vi "save_testConditions.vi"(8 "error in (no error)":errorcluster, 11 "cmd":T5) -> (0 "error out":errorcluster)   [LabVIEW 2019]
uses:
  cmd_TestParaSave.ctl
  type_testpara.ctl
  Capacitor/cap_config.ctl
  Capacitor/Judge_RC.ctl
  _ctrl/rw.ctl
  Global_params.vi
  Global 1.vi
  <vilib>/Utility/xml.llb/Write to XML File(string).vi
  <vilib>/Utility/xml.llb/Read From XML File(string).vi
  SubVIs/common/Glob_Ref.vi
panel:
  out "Test Mode":T1
  out "RC-Testconfig.Test Mode":T1
  out "TestConditons":T2={"Breakdown-Spec"={"제어단 단선 Irms[mA](이하)"=0.0, "제어단 특성 전류 Irms[mA] Max"=0.0, "제어단 특성 전류 Irms[mA] Min"=0.0, "출력단 단선 Irms[mA](이하)"=0.0, "출력단 특성 전류 Irms[mA]  Max"=0.0, "출력단 특성전류 Irms[mA]  Min"=0.0, "온도[degree]"=0.0}, "RC-Testconfig"={"Test Mode"=enum."6.3.2 저온 작동/방치 시험", "ON time[ms]"=500.0, "OFF time[ms]"=500.0, "1. 작동시간[분]"=10000.0, "2. 미작동시간[분]"=10000.0, "3. 작동시간[분]"=10000.0, "level[V]"=12.0, "duty"=20.0, "Freq"=1.0, "Voltage+[V]"=20.0, "Voltage-[V]"=-20.0, "Current+[A]"=5.0, "Current-[A]"=-5.0, "출력전압[V]"=0.0, "출력전류[A]"=0.0, "OVP Level"=0.0, "OCP Level"=0.0, "Time Div"=7, "Record Len"=4, "방전 기준[V]"=0.0, "Repeate (Each Ch)"=1, "Cycle[N]"=1, "작동간격[분]"=10000.0, "TrigPos[%]"=0.0, "시험시간[분]"=1.0}, "RC-Test Judgement "={"전압 63%[mS] Min"=0.0, "전압 98%[mS] Min"=0.0, "전류 37%[mS] Min"=0.0, "접촉저항[mOhm] Min"=0.0, "출력전류 Irms[mA] Min"=0.0, "전압 63%[mS] Max"=0.0, "전압 98%[mS] Max"=0.0, "전류 37%[mS] Max"=0.0, "접촉저항[mOhm] Max"=0.0, "출력전류 Irms[mA] Max"=0.0}, "Log path"=path "", "file renew[Hr]"=0, "시험명"="R", "시험모드 선택"=enum."6.3.2 저온 작동/방치 시험"} {"RC-Testconfig"."시험시간[분]" min=1.0; "RC-Testconfig"."작동간격[분]" min=1.0; "RC-Testconfig"."3. 작동시간[분]" min=1.0; "RC-Testconfig"."2. 미작동시간[분]" min=1.0; "RC-Testconfig"."1. 작동시간[분]" min=1.0; "RC-Testconfig"."Time Div" items=["10m", "20ms", "50ms", "100ms", "200ms", "500ms", "1s", "2s", "5s", "10s", "20s", "30s", "1min", "2min", "5min"]; "RC-Testconfig"."OFF time[ms]" min=10000.0 max=1000000.0; "RC-Testconfig"."Current-[A]" min=-20.0 max=20.0 step=0.001; "RC-Testconfig"."Voltage-[V]" min=-115.0 max=115.0 step=0.01; "RC-Testconfig"."Current+[A]" min=0.0 max=60.0 step=0.01; "RC-Testconfig"."Voltage+[V]" min=0.0 max=120.0 step=0.1; "RC-Testconfig"."OCP Level" format="%#_13g"; "RC-Testconfig"."OVP Level" format="%#_13g"; "RC-Testconfig"."Record Len" items=["10k", "25k", "50k", "100k", "250k", "500k", "1M", "2.5M", "5M", "10M", "25M", "50M", "100M", "250M", "500M", "1G", "2G", "4G", "5G", "10G", "20G", "50G"]; "RC-Testconfig"."ON time[ms]" min=50.0 max=2000000.0}
  # "제어단"
  # "출력단"
  # "온도기준"
  # "제어단 전압"
  # "출력단 전원"
  # "DL950"
  # "Discharge"
  # "Test Cycle"
  # "작동 설정"
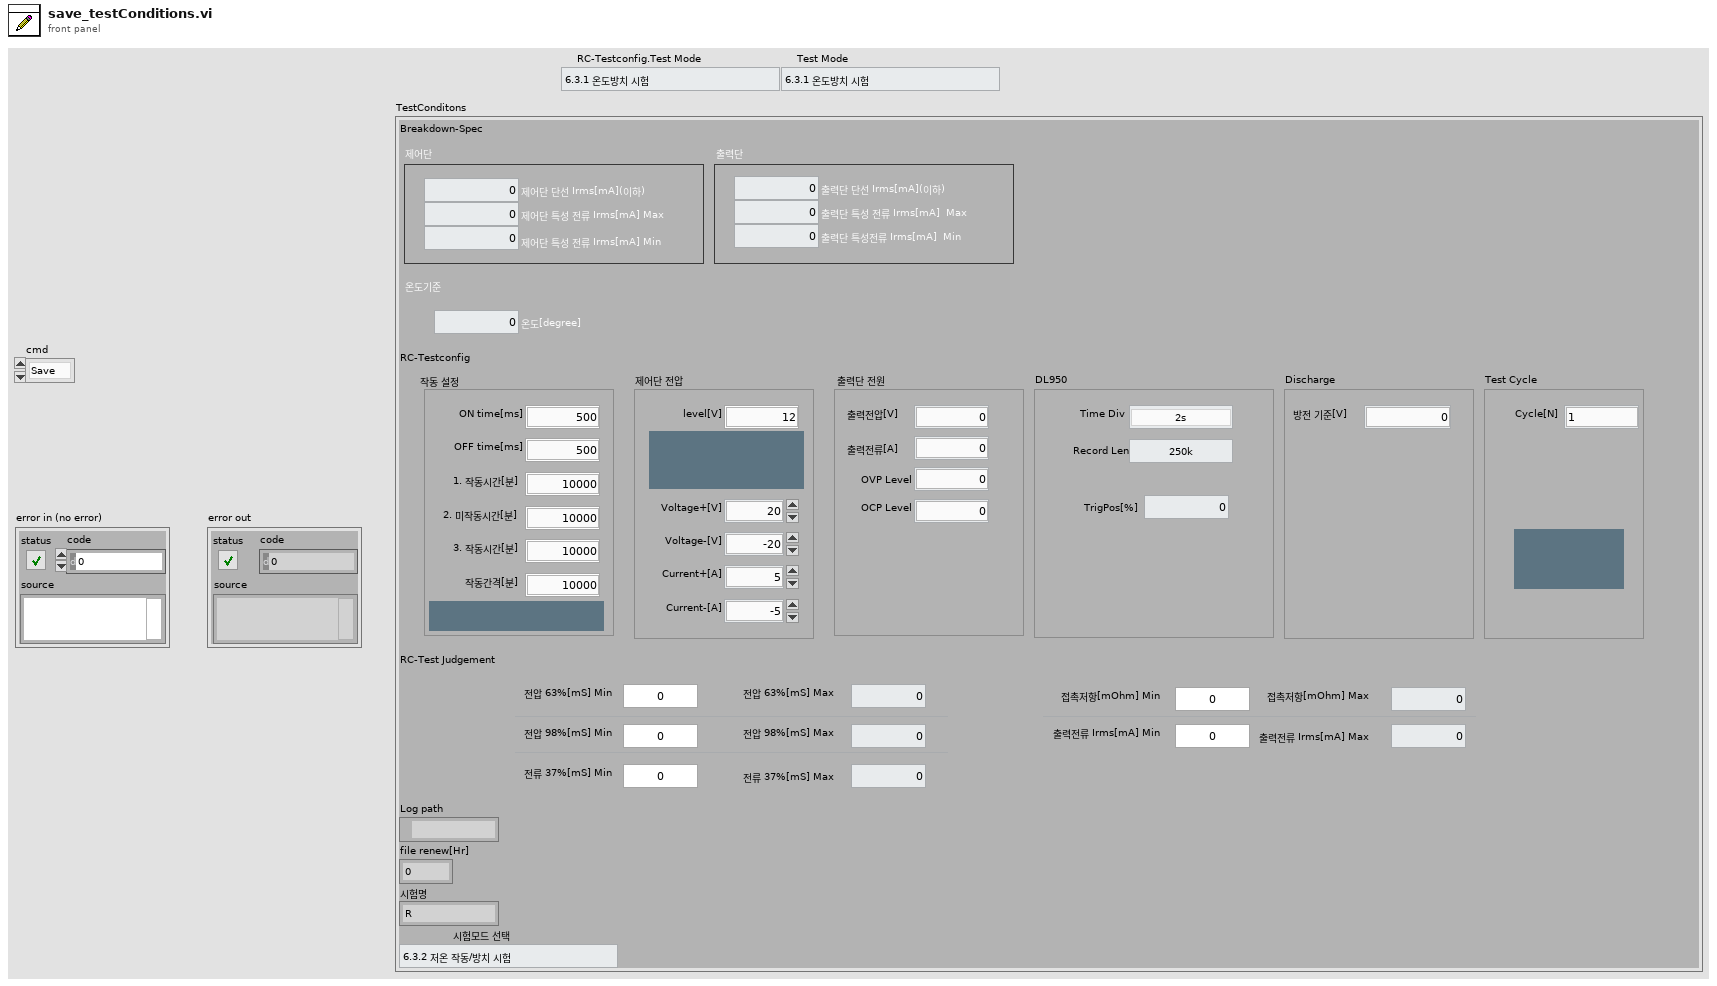
[diagram p1: front panel]
types:
  T1 = typedef "시험모드선택.ctl" = enum16{"6.3.1 온도방치 시험", "6.3.2 저온 작동/방치 시험", "6.3.3 고온 작동/방치 시험", "6.3.4 온도 싸이클 시험", "6.3.6 온습도 싸이클 시험", "6.3.7 고온고습 방치", "6.3.8 결로 시험", "6.3.9 빙결시험", "6.3.10 공진", "6.3.11.1 작동가진", "6.3.11.2 비작동 가진 ", "6.3.12 충격시험"}
  T2 = typedef "type_testpara.ctl" = cluster{"Breakdown-Spec":cluster{"제어단 단선 Irms[mA](이하)":dbl, "제어단 특성 전류 Irms[mA] Max":dbl, "제어단 특성 전류 Irms[mA] Min":dbl, "출력단 단선 Irms[mA](이하)":dbl, "출력단 특성 전류 Irms[mA]  Max":dbl, "출력단 특성전류 Irms[mA]  Min":dbl, "온도[degree]":dbl}, "RC-Testconfig":T3, "RC-Test Judgement ":T4, "Log path":path, "file renew[Hr]":u8, "시험명":string, "시험모드 선택":T1}
  T3 = typedef "cap_config.ctl" = cluster{"Test Mode":T1, "ON time[ms]":dbl, "OFF time[ms]":dbl, "1. 작동시간[분]":dbl, "2. 미작동시간[분]":dbl, "3. 작동시간[분]":dbl, "level[V]":dbl, "duty":dbl, "Freq":dbl, "Voltage+[V]":dbl, "Voltage-[V]":dbl, "Current+[A]":dbl, "Current-[A]":dbl, "출력전압[V]":dbl, "출력전류[A]":dbl, "OVP Level":dbl, "OCP Level":dbl, "Time Div":u16, "Record Len":i32, "방전 기준[V]":dbl, "Repeate (Each Ch)":u32, "Cycle[N]":u32, "작동간격[분]":dbl, "TrigPos[%]":dbl, "시험시간[분]":dbl}
  T4 = typedef "Judge_RC.ctl" = cluster{"전압 63%[mS] Min":dbl, "전압 98%[mS] Min":dbl, "전류 37%[mS] Min":dbl, "접촉저항[mOhm] Min":dbl, "출력전류 Irms[mA] Min":dbl, "전압 63%[mS] Max":dbl, "전압 98%[mS] Max":dbl, "전류 37%[mS] Max":dbl, "접촉저항[mOhm] Max":dbl, "출력전류 Irms[mA] Max":dbl}
  T5 = typedef "cmd_TestParaSave.ctl" = enum16{"Save", "Read", "Idle"}
  T6 = typedef "rw.ctl" = enum16{"read", "write"}
  T7 = enum16{"open", "replace", "create", "open or create", "replace or create", "replace or create with confirmation"}
  T8 = enum8{"Enabled", "Disabled", "Disabled and Grayed Out"}
  T9 = enum32{"6.3.2 저온 작동/방치 시험", "6.3.3 고온 작동/방치 시험", "6.3.4 온도 싸이클 시험", "6.3.6 온습도 싸이클 시험", "6.3.8 결로 시험", "6.3.9 빙결 시험"}
  T10 = cluster{"Freq":dbl, "level[V]":dbl, "duty":dbl, "On time[ms]":dbl}
  T11 = typedef "Test Mode.ctl" = enum32{"저항부하", "캐패시터부하", "B수명 - 1", "B수명 - 2", "B수명 - 3", "저전압모드 동작검사", "저전압모드 접촉저항", "고전압모드 동작검사"}
  T12 = typedef "ref_all.ctl" = cluster{"BP4610 Config":refnum<vi>, "DSP1950 Config":refnum<vi>, "2470-config":refnum<vi>, "cDAQ 9269 AO config":refnum<vi>, "cDAQ 9221 Config":refnum<vi>, "cDAQ-9467 Config":refnum<vi>, "Waveform":refnum<vi>, "DL950 wfm":refnum<vi>, "AI Graph":refnum<vi>, "AO_Wave-config":refnum<vi>, "DL950 items":refnum<vi>, "Volt":refnum<vi>, "Current":refnum<vi>, "AO_Level":refnum<vi>, "RC-Test Judgement ":refnum<vi>, "Log path":refnum<vi>, "시험명":refnum<vi>, "file renew[Hr]":refnum<vi>, "Breakdown-Spec":refnum<vi>, "paste":refnum<vi>, "copy":refnum<vi>, "DL950_config":refnum<vi>, "종료시간":refnum<vi>, "경과시간":refnum<vi>, "Apply":refnum<vi>, "DSP Config LV ":refnum<vi>, "Testconfig":refnum<vi>}
  T13 = typedef "Breakdown-Spec.ctl" = cluster{"제어단 단선 Irms[mA](이하)":dbl, "제어단 특성 전류 Irms[mA] Max":dbl, "제어단 특성 전류 Irms[mA] Min":dbl, "출력단 단선 Irms[mA](이하)":dbl, "출력단 특성 전류 Irms[mA]  Max":dbl, "출력단 특성전류 Irms[mA]  Min":dbl, "온도[degree]":dbl}
  T14 = cluster{"제어단 단선 Irms[mA](이하)":dbl, "제어단 특성 전류 Irms[mA] Max":dbl, "제어단 특성 전류 Irms[mA] Min":dbl, "출력단 단선 Irms[mA](이하)":dbl, "출력단 특성 전류 Irms[mA]  Max":dbl, "출력단 특성전류 Irms[mA]  Min":dbl, "온도[degree]":dbl}
  T15 = enum8{"Enabled", "Disabled", "Disabled and Grayed Out"}[]
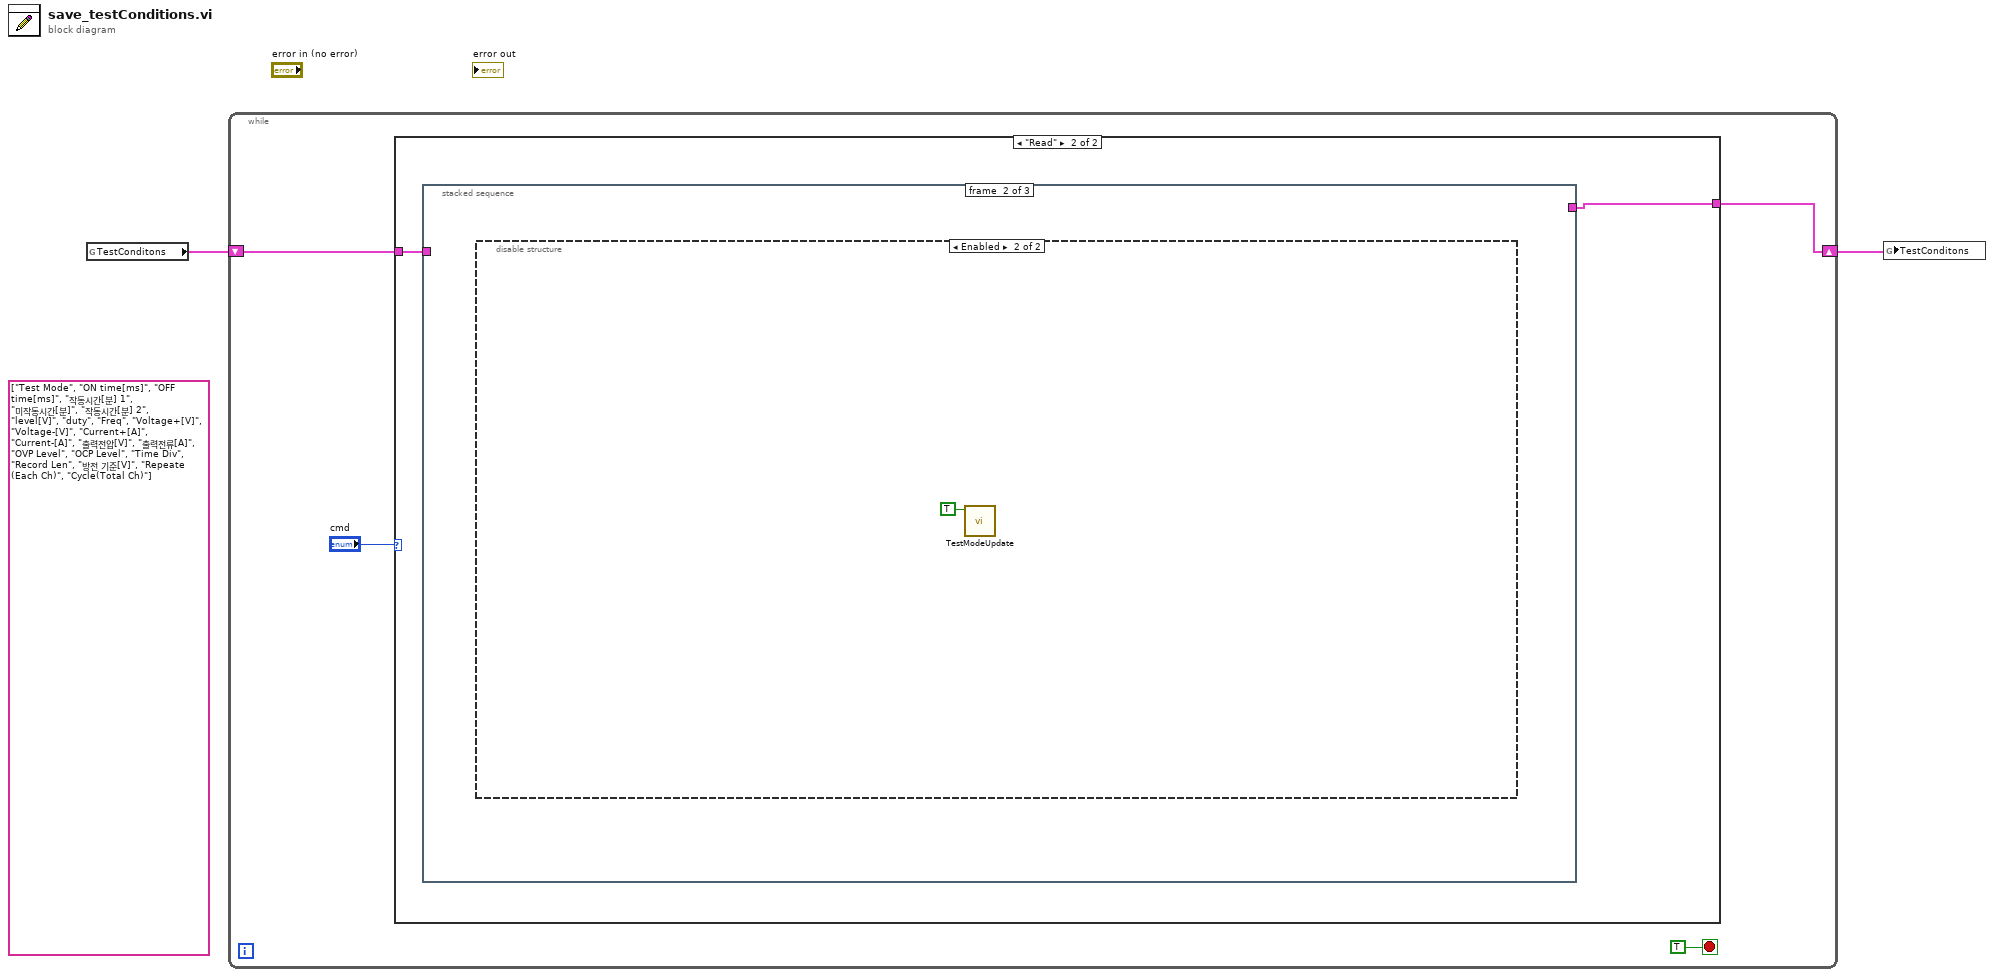
[diagram p0: block diagram]
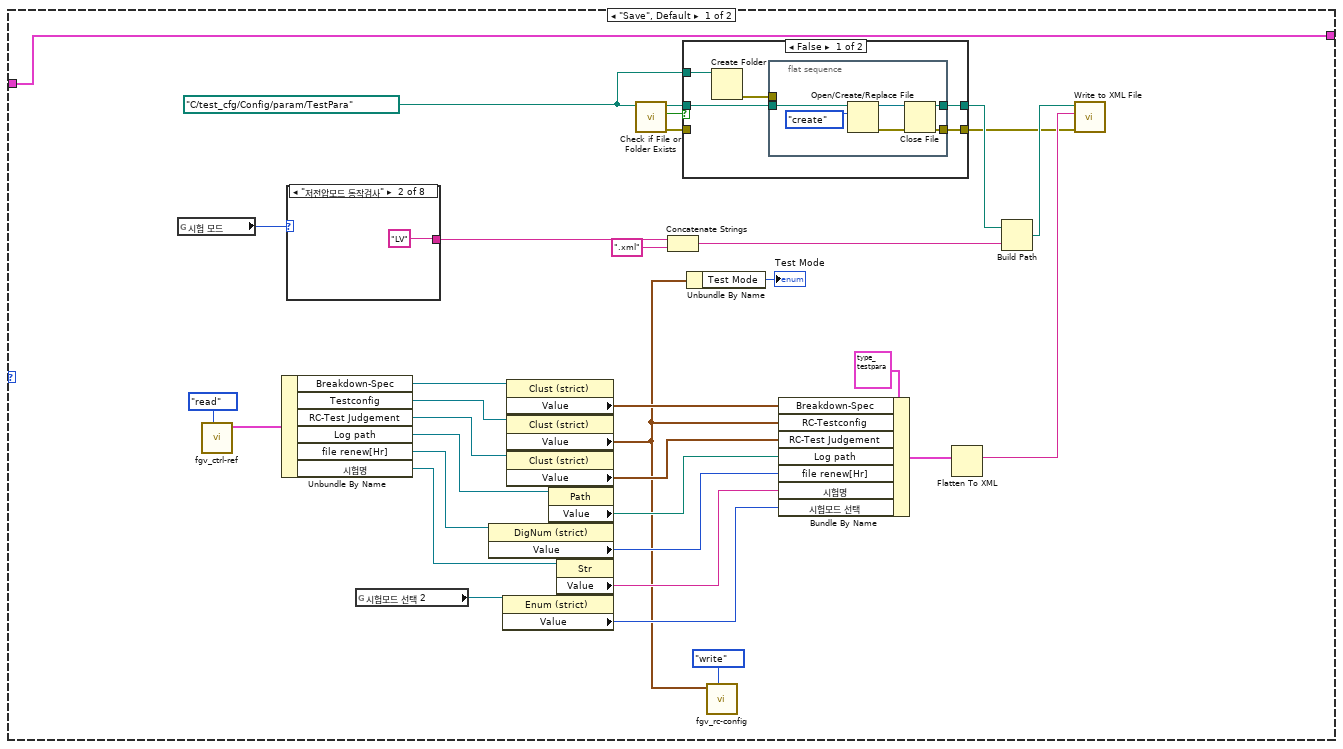
[diagram p2: hidden frame]
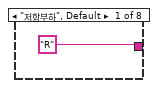
[diagram p3: hidden frame]
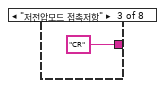
[diagram p4: hidden frame]
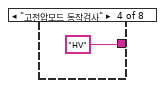
[diagram p5: hidden frame]
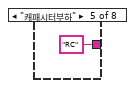
[diagram p6: hidden frame]
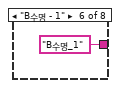
[diagram p7: hidden frame]
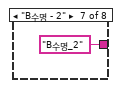
[diagram p8: hidden frame]
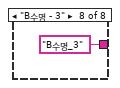
[diagram p9: hidden frame]
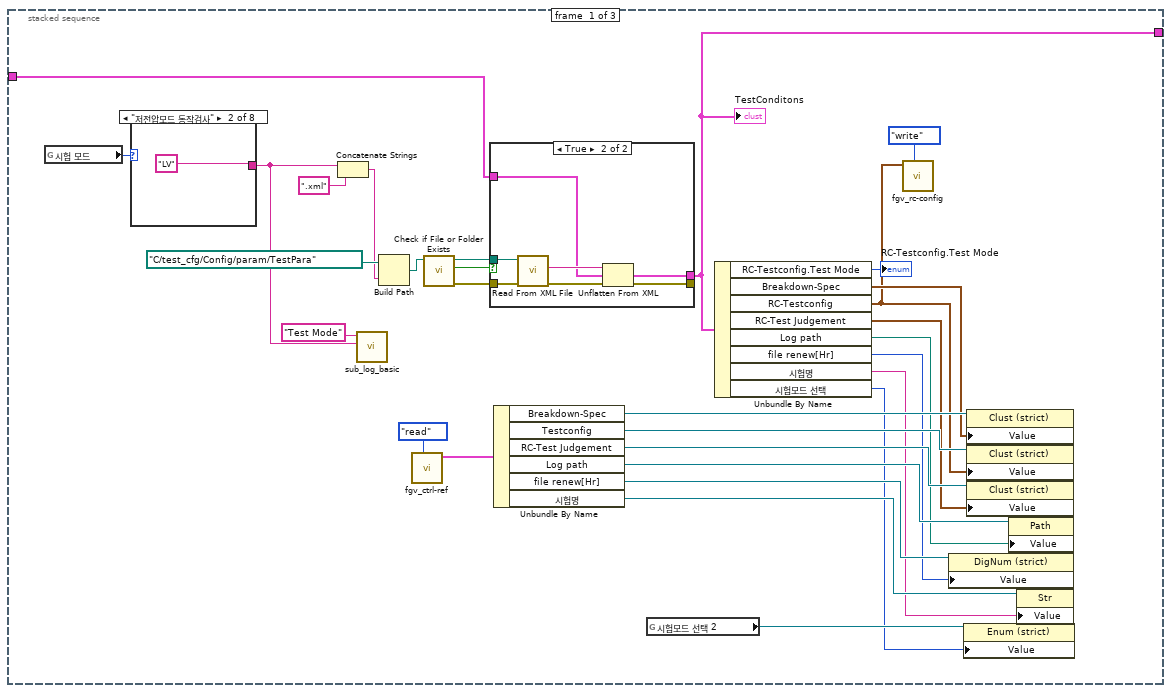
[diagram p11: hidden frame]
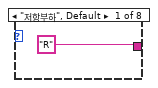
[diagram p13: hidden frame]
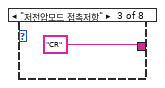
[diagram p14: hidden frame]
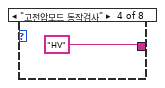
[diagram p15: hidden frame]
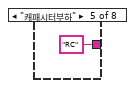
[diagram p16: hidden frame]
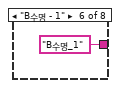
[diagram p17: hidden frame]
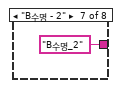
[diagram p18: hidden frame]
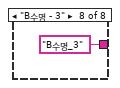
[diagram p19: hidden frame]
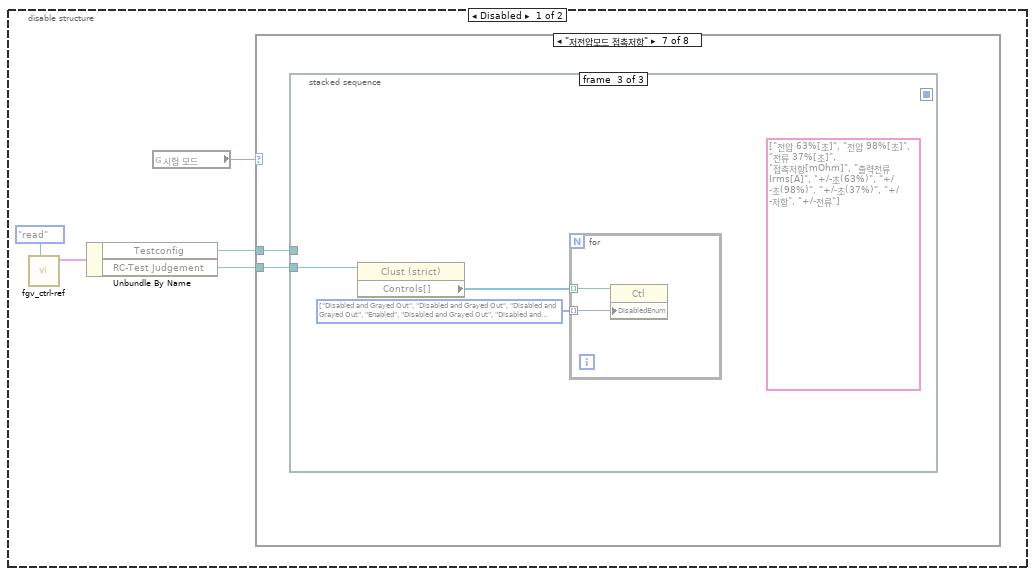
[diagram p20: hidden frame]
diagram:
  (unwired) string[] ["Test Mode", "ON time[ms]", "OFF time[ms]", "작동시간[분] 1", "미작동시간[분]", "작동시간[분] 2", "level[V]", "duty", "Freq", "Voltage+[V]", "Voltage-[V]", "Current+[A]", "Current-[A]", "출력전압[V]", "출력전류[A]", "OVP Level", "OCP Level", "Time Div", "Record Len", "방전 기준[V]", "Repeate (Each Ch)", "Cycle(Total Ch)"] ("Array 2")
  n1 = global read "Global_params.vi" "TestConditons"() -> (w2:T2)
  n2 = while {
    shift-right: [w3] -> w1
    shift-left: w2 -> [w4]
    stop <- TRUE stop-if-true
    n3 = case shown="\"Read\"" "cmd" {
      tunnel: w4 -> [w15 w62]
      tunnel: [w15 w61] -> w3
      frame "Save", Default {
        w14 = path "C:/test_cfg/Config/param/TestPara" ("XML File Path")
        n4 = global read "Global 1.vi" "시험 모드"() -> (w13:T11)
        n5 = call "fgv_ctrl-ref.vi"("cmd"=rw."read") -> ("output cluster 2"=w38:T12)  [unwired: 9 in, 1 out]
        n6 = Unbundle By Name(w38) -> ("Breakdown-Spec"=w37:refnum<vi>, "Testconfig"=w36:refnum<vi>, "RC-Test Judgement"=w35:refnum<vi>, "Log path"=w34:refnum<vi>, "file renew[Hr]"=w33:refnum<vi>, "시험명"=w32:refnum<vi>)
        n7 = case shown="\"저전압모드 동작검사\"" w13 {
          tunnel: ["R" "LV" "CR" "HV" "RC" "B수명_1" "B수명_2" "B수명_3"] -> w12
          frame "저항부하", Default {
          }
          frame "저전압모드 동작검사" {
          }
          frame "저전압모드 접촉저항" {
          }
          frame "고전압모드 동작검사" {
          }
          frame "캐패시터부하" {
          }
          frame "B수명 - 1" {
          }
          frame "B수명 - 2" {
          }
          frame "B수명 - 3" {
          }
        }
        n8 = global read "Global 1.vi" "시험모드 선택 2"() -> (w10:refnum<vi>)
        n9 = property class="DigNum (strict)"(reference=w33) -> ("Value"=w28:i32)  [unwired: 1 in, 2 out]
        n10 = property class="Enum (strict)"(reference=w10) -> ("Value"=w9:T1)  [unwired: 1 in, 2 out]
        n11 = property class="Clust (strict)"(reference=w37) -> ("Value"=w26:T13)  [unwired: 1 in, 2 out]
        n12 = property class="Clust (strict)"(reference=w36) -> ("Value"=w8:T3)  [unwired: 1 in, 2 out]
        n13 = property class="Clust (strict)"(reference=w35) -> ("Value"=w30:T4)  [unwired: 1 in, 2 out]
        n14 = property class="Path"(reference=w34) -> ("Value"=w29:path)  [unwired: 1 in, 2 out]
        n15 = property class="Str"(reference=w32) -> ("Value"=w27:string)  [unwired: 1 in, 2 out]
        n16 = call <vilib>:"Check if File or Folder Exists.vi"("path"=w14) -> ("error out"=w23:errorcluster, "file or folder exists?"=w25:bool, "dup path"=w24:path)  [unwired: 8 in]
        n17 = Concatenate Strings(w12, ".xml" ("문자열")) -> (w18:string)
        n18 = case shown="False" w25 {
          tunnel: w23 -> [_ w60]
          tunnel: w24 -> [w52 w59]
          tunnel: [w50 w60] -> w16
          tunnel: [w51 w59] -> w20
          tunnel: w14 -> [w49 _]
          frame False {
            n19 = Create Folder(path (use dialog)=w49) -> (error out=w48:errorcluster)  [unwired: 2 in, 2 out]
            n20 = flat-sequence {
              tunnel: w52 -> [w58]
              tunnel: [w54] -> w51
              tunnel: [w53] -> w50
              tunnel: w48 -> [_]
              frame #0 {
                n21 = Open/Create/Replace File(file path (use dialog)=w58, operation (0:open)=T7."create" ("동작(0:open)")) -> (refnum out=w55:refnum<file>, error out=w56:errorcluster)  [unwired: 4 in, 1 out]
                n22 = Close File(refnum=w55, error in=w56) -> (path=w54:path, error out=w53:errorcluster)
              }
            }
          }
          frame True {
          }
        }
        n23 = Unbundle By Name(w8) -> ("Test Mode"=→"Test Mode":T1)
        n24 = call "fgv_rc-config.vi"("cmd"=rw."write", "Testconfig"=w8) -> ()  [unwired: 8 in, 2 out]
        n25 = Bundle By Name(cluster=T2 {"Breakdown-Spec"={"제어단 단선 Irms[mA](이하)"=0.0, "제어단 특성 전류 Irms[mA] Max"=0.0, "제어단 특성 전류 Irms[mA] Min"=0.0, "출력단 단선 Irms[mA](이하)"=0.0, "출력단 특성 전류 Irms[mA]  Max"=0.0, "출력단 특성전류 Irms[mA]  Min"=0.0, "온도[degree]"=0.0}, "RC-Testconfig"={"Test Mode"=enum."6.3.2 저온 작동/방치 시험", "ON time[ms]"=500.0, "OFF time[ms]"=500.0, "1. 작동시간[분]"=10000.0, "2. 미작동시간[분]"=10000.0, "3. 작동시간[분]"=10000.0, "level[V]"=12.0, "duty"=20.0, "Freq"=1.0, "Voltage+[V]"=20.0, "Voltage-[V]"=-20.0, "Current+[A]"=5.0, "Current-[A]"=-5.0, "출력전압[V]"=0.0, "출력전류[A]"=0.0, "OVP Level"=0.0, "OCP Level"=0.0, "Time Div"=7, "Record Len"=4, "방전 기준[V]"=0.0, "Repeate (Each Ch)"=1, "Cycle[N]"=1, "작동간격[분]"=10000.0, "TrigPos[%]"=0.0, "시험시간[분]"=1.0}, "RC-Test Judgement "={"전압 63%[mS] Min"=0.0, "전압 98%[mS] Min"=0.0, "전류 37%[mS] Min"=0.0, "접촉저항[mOhm] Min"=0.0, "출력전류 Irms[mA] Min"=0.0, "전압 63%[mS] Max"=0.0, "전압 98%[mS] Max"=0.0, "전류 37%[mS] Max"=0.0, "접촉저항[mOhm] Max"=0.0, "출력전류 Irms[mA] Max"=0.0}, "Log path"=path "", "file renew[Hr]"=0, "시험명"="R", "시험모드 선택"=enum."6.3.2 저온 작동/방치 시험"} ("Cluster"), "Breakdown-Spec"=w26, "RC-Testconfig"=w8, "RC-Test Judgement"=w30, "Log path"=w29, "file renew[Hr]"=w28, "시험명"=w27, "시험모드 선택"=w9) -> (w21:T2)
        n26 = Flatten To XML(anything=w21) -> (xml string=w22:string)
        n27 = Build Path(base path=w20, name or relative path=w18) -> (appended path=w17:path)
        n28 = call-poly <vilib>:"Write to XML File.vi"("error in (no error)"=w16, "XML Input"=w22, "XML File Path"=w17) -> ()  [unwired: 6 in, 3 out]
      }
      frame "Read" {
        n29 = stacked-sequence {
          tunnel: w62 -> [w86 _ _]
          tunnel: [w75 _ _] -> w61
          frame #0 {
            n30 = global read "Global 1.vi" "시험 모드"() -> (w92:T11)
            n31 = case shown="\"저전압모드 동작검사\"" w92 {
              tunnel: ["R" "LV" "CR" "HV" "RC" "B수명_1" "B수명_2" "B수명_3"] -> w66
              frame "저항부하", Default {
              }
              frame "저전압모드 동작검사" {
              }
              frame "저전압모드 접촉저항" {
              }
              frame "고전압모드 동작검사" {
              }
              frame "캐패시터부하" {
              }
              frame "B수명 - 1" {
              }
              frame "B수명 - 2" {
              }
              frame "B수명 - 3" {
              }
            }
            n32 = Concatenate Strings(w66, ".xml" ("문자열")) -> (w85:string)
            n33 = call "sub_log_basic.vi"("desc"=w66, "Title"="Test Mode") -> ()  [unwired: 9 in, 1 out]
            n34 = Build Path(base path=path "C:/test_cfg/Config/param/TestPara" ("XML File Path"), name or relative path=w85) -> (appended path=w84:path)
            n35 = call "fgv_ctrl-ref.vi"("cmd"=rw."read") -> ("output cluster 2"=w82:T12)  [unwired: 9 in, 1 out]
            n36 = call <vilib>:"Check if File or Folder Exists.vi"("path"=w84) -> ("error out"=w88:errorcluster, "file or folder exists?"=w89:bool, "dup path"=w90:path)  [unwired: 8 in]
            n37 = case shown="True" w89 {
              tunnel: w86 -> [_ w99]
              tunnel: [_ w98] -> w75
              tunnel: [w93 w96] -> _
              tunnel: w90 -> [_ w95]
              tunnel: w88 -> [w93 w94]
              frame False {
              }
              frame True {
                n38 = call-poly <vilib>:"Read From XML File.vi"("error in (no error)"=w94, "XML File Path"=w95) -> ("error out"=w97:errorcluster, "XML Elements"=w100:string)  [unwired: 7 in, 1 out]
                n39 = Unflatten From XML(xml string=w100, type=w99, error in (no error)=w97) -> (value=w98:T2, error out=w96:errorcluster)
              }
            }
            "TestConditons" <- w75
            n40 = Unbundle By Name(w82) -> ("Breakdown-Spec"=w81:refnum<vi>, "Testconfig"=w80:refnum<vi>, "RC-Test Judgement"=w79:refnum<vi>, "Log path"=w78:refnum<vi>, "file renew[Hr]"=w77:refnum<vi>, "시험명"=w76:refnum<vi>)
            n41 = global read "Global 1.vi" "시험모드 선택 2"() -> (w65:refnum<vi>)
            n42 = Unbundle By Name(w75) -> ("RC-Testconfig.Test Mode"=→"RC-Testconfig.Test Mode":T1, "Breakdown-Spec"=w74:T14, "RC-Testconfig"=w69:T3, "RC-Test Judgement"=w73:T4, "Log path"=w72:path, "file renew[Hr]"=w71:u8, "시험명"=w70:string, "시험모드 선택"=w64:T1)
            n43 = call "fgv_rc-config.vi"("cmd"=rw."write", "Testconfig"=w69) -> ()  [unwired: 8 in, 2 out]
            n44 = property class="DigNum (strict)"(reference=w77, "Value"=w71) -> ()  [unwired: 1 in, 2 out]
            n45 = property class="Enum (strict)"(reference=w65, "Value"=w64) -> ()  [unwired: 1 in, 2 out]
            n46 = property class="Clust (strict)"(reference=w81, "Value"=w74) -> ()  [unwired: 1 in, 2 out]
            n47 = property class="Clust (strict)"(reference=w80, "Value"=w69) -> ()  [unwired: 1 in, 2 out]
            n48 = property class="Clust (strict)"(reference=w79, "Value"=w73) -> ()  [unwired: 1 in, 2 out]
            n49 = property class="Path"(reference=w78, "Value"=w72) -> ()  [unwired: 1 in, 2 out]
            n50 = property class="Str"(reference=w76, "Value"=w70) -> ()  [unwired: 1 in, 2 out]
          }
          frame #1 {
            n51 = disable-structure shown="Enabled" {
              frame Disabled {
                n52 = call "fgv_ctrl-ref.vi"("cmd"=rw."read") -> ("output cluster 2"=w112:T12)  [unwired: 9 in, 1 out]
                n53 = Unbundle By Name(w112) -> ("Testconfig"=w110:refnum<vi>, "RC-Test Judgement"=w109:refnum<vi>)
                n54 = global read "Global 1.vi" "시험 모드"() -> (w111:T11)
                n55 = case shown="\"저전압모드 접촉저항\"" w111 {
                  tunnel: w110 -> [w115 w127 w139 w151 w163 w175 w197 w222]
                  tunnel: w109 -> [w114 w126 w138 w150 w162 w174 w196 w221]
                  frame "저항부하", Default {
                    n56 = stacked-sequence {
                      tunnel: w115 -> [w120 _]
                      tunnel: w114 -> [_ w123]
                      frame #0 {
                        (unwired) string[] ["출력전압[V]", "출력전류[A]", "방전 기준[V]", "Freq", "level[V]", "duty", "On time[ms]", "Record Len", "Time Div", "Repeate", "Test Cycle"] ("Array")
                        n57 = property class="Clust (strict)"(reference=w120) -> ("Controls[]"=w118:refnum<vi>[])  [unwired: 1 in, 2 out]
                        n58 = Index Array(array=w118, index=2) -> (element=w116:refnum<vi>)
                        n59 = property class="Ctl" props=["Label", "Text", "DisabledEnum"](reference=w116, "DisabledEnum"=T8."Disabled and Grayed Out" ("Disabled")) -> ()  [unwired: 1 in, 3 out]
                      }
                      frame #1 {
                        w121 = T15 [enum."Disabled and Grayed Out", enum."Disabled and Grayed Out", enum."Disabled and Grayed Out", enum."Disabled and Grayed Out", enum."Enabled", enum."Disabled and Grayed Out", enum."Disabled and Grayed Out", enum."Disabled and Grayed Out", enum."Disabled and Grayed Out", enum."Enabled"] items=["Enabled", "Disabled", "Disabled and Grayed Out"]
                        (unwired) string[] ["전압 63%[초]", "전압 98%[초]", "전류 37%[초]", "접촉저항[mOhm]", "출력전류 Irms[A]", "+/-초(63%)", "+/-초(98%)", "+/-초(37%)", "+/-저항", "+/-전류"] ("Array")
                        n60 = property class="Clust (strict)"(reference=w123) -> ("Controls[]"=w122:refnum<vi>[])  [unwired: 1 in, 2 out]
                        n61 = for {
                          tunnel: w122 -> [w125] mode=indexing
                          tunnel: w121 -> [w124] mode=indexing
                          n62 = property class="Ctl"(reference=w125, "DisabledEnum"=w124) -> ()  [unwired: 1 in, 2 out]
                        }
                      }
                    }
                  }
                  frame "캐패시터부하" {
                    n63 = stacked-sequence {
                      tunnel: w127 -> [w132 _]
                      tunnel: w126 -> [_ w135]
                      frame #0 {
                        n64 = property class="Clust (strict)"(reference=w132) -> ("Controls[]"=w130:refnum<vi>[])  [unwired: 1 in, 2 out]
                        n65 = Index Array(array=w130, index=2) -> (element=w128:refnum<vi>)
                        n66 = property class="Ctl" props=["Label", "Text", "DisabledEnum"](reference=w128, "DisabledEnum"=T8."Enabled" ("Disabled")) -> ()  [unwired: 1 in, 3 out]
                      }
                      frame #1 {
                        w133 = T15 [enum."Enabled", enum."Enabled", enum."Enabled", enum."Enabled", enum."Enabled", enum."Enabled", enum."Enabled", enum."Enabled", enum."Enabled", enum."Enabled"] items=["Enabled", "Disabled", "Disabled and Grayed Out"]
                        n67 = property class="Clust (strict)"(reference=w135) -> ("Controls[]"=w134:refnum<vi>[])  [unwired: 1 in, 2 out]
                        n68 = for {
                          tunnel: w134 -> [w137] mode=indexing
                          tunnel: w133 -> [w136] mode=indexing
                          n69 = property class="Ctl"(reference=w137, "DisabledEnum"=w136) -> ()  [unwired: 1 in, 2 out]
                        }
                      }
                    }
                  }
                  frame "B수명 - 1" {
                    n70 = stacked-sequence {
                      tunnel: w139 -> [w144 _]
                      tunnel: w138 -> [_ w147]
                      frame #0 {
                        (unwired) string[] ["출력전압[V]", "출력전류[A]", "방전 기준[V]", "Freq", "level[V]", "duty", "On time[ms]", "Record Len", "Time Div", "Repeate", "Test Cycle"] ("Array")
                        n71 = property class="Clust (strict)"(reference=w144) -> ("Controls[]"=w142:refnum<vi>[])  [unwired: 1 in, 2 out]
                        n72 = Index Array(array=w142, index=2) -> (element=w140:refnum<vi>)
                        n73 = property class="Ctl" props=["Label", "Text", "DisabledEnum"](reference=w140, "DisabledEnum"=T8."Enabled" ("Disabled")) -> ()  [unwired: 1 in, 3 out]
                      }
                      frame #1 {
                        w145 = T15 [enum."Enabled", enum."Enabled", enum."Enabled", enum."Enabled", enum."Enabled", enum."Enabled", enum."Enabled", enum."Enabled", enum."Enabled", enum."Enabled"] items=["Enabled", "Disabled", "Disabled and Grayed Out"]
                        (unwired) string[] ["전압 63%[초]", "전압 98%[초]", "전류 37%[초]", "접촉저항[mOhm]", "출력전류 Irms[A]", "+/-초(63%)", "+/-초(98%)", "+/-초(37%)", "+/-저항", "+/-전류"] ("Array")
                        n74 = property class="Clust (strict)"(reference=w147) -> ("Controls[]"=w146:refnum<vi>[])  [unwired: 1 in, 2 out]
                        n75 = for {
                          tunnel: w146 -> [w149] mode=indexing
                          tunnel: w145 -> [w148] mode=indexing
                          n76 = property class="Ctl"(reference=w149, "DisabledEnum"=w148) -> ()  [unwired: 1 in, 2 out]
                        }
                      }
                    }
                  }
                  frame "B수명 - 2" {
                    n77 = stacked-sequence {
                      tunnel: w151 -> [w156 _]
                      tunnel: w150 -> [_ w159]
                      frame #0 {
                        (unwired) string[] ["출력전압[V]", "출력전류[A]", "방전 기준[V]", "Freq", "level[V]", "duty", "On time[ms]", "Record Len", "Time Div", "Repeate", "Test Cycle"] ("Array")
                        n78 = property class="Clust (strict)"(reference=w156) -> ("Controls[]"=w154:refnum<vi>[])  [unwired: 1 in, 2 out]
                        n79 = Index Array(array=w154, index=2) -> (element=w152:refnum<vi>)
                        n80 = property class="Ctl" props=["Label", "Text", "DisabledEnum"](reference=w152, "DisabledEnum"=T8."Disabled and Grayed Out" ("Disabled")) -> ()  [unwired: 1 in, 3 out]
                      }
                      frame #1 {
                        w157 = T15 [enum."Disabled and Grayed Out", enum."Disabled and Grayed Out", enum."Disabled and Grayed Out", enum."Disabled and Grayed Out", enum."Enabled", enum."Disabled and Grayed Out", enum."Disabled and Grayed Out", enum."Disabled and Grayed Out", enum."Disabled and Grayed Out", enum."Enabled"] items=["Enabled", "Disabled", "Disabled and Grayed Out"]
                        (unwired) string[] ["전압 63%[초]", "전압 98%[초]", "전류 37%[초]", "접촉저항[mOhm]", "출력전류 Irms[A]", "+/-초(63%)", "+/-초(98%)", "+/-초(37%)", "+/-저항", "+/-전류"] ("Array")
                        n81 = property class="Clust (strict)"(reference=w159) -> ("Controls[]"=w158:refnum<vi>[])  [unwired: 1 in, 2 out]
                        n82 = for {
                          tunnel: w158 -> [w161] mode=indexing
                          tunnel: w157 -> [w160] mode=indexing
                          n83 = property class="Ctl"(reference=w161, "DisabledEnum"=w160) -> ()  [unwired: 1 in, 2 out]
                        }
                      }
                    }
                  }
                  frame "B수명 - 3" {
                    n84 = stacked-sequence {
                      tunnel: w163 -> [w168 _]
                      tunnel: w162 -> [_ w171]
                      frame #0 {
                        (unwired) string[] ["출력전압[V]", "출력전류[A]", "방전 기준[V]", "Freq", "level[V]", "duty", "On time[ms]", "Record Len", "Time Div", "Repeate", "Test Cycle"] ("Array")
                        n85 = property class="Clust (strict)"(reference=w168) -> ("Controls[]"=w166:refnum<vi>[])  [unwired: 1 in, 2 out]
                        n86 = Index Array(array=w166, index=2) -> (element=w164:refnum<vi>)
                        n87 = property class="Ctl" props=["Label", "Text", "DisabledEnum"](reference=w164, "DisabledEnum"=T8."Disabled and Grayed Out" ("Disabled")) -> ()  [unwired: 1 in, 3 out]
                      }
                      frame #1 {
                        w169 = T15 [enum."Disabled and Grayed Out", enum."Disabled and Grayed Out", enum."Disabled and Grayed Out", enum."Disabled and Grayed Out", enum."Enabled", enum."Disabled and Grayed Out", enum."Disabled and Grayed Out", enum."Disabled and Grayed Out", enum."Disabled and Grayed Out", enum."Enabled"] items=["Enabled", "Disabled", "Disabled and Grayed Out"]
                        (unwired) string[] ["전압 63%[초]", "전압 98%[초]", "전류 37%[초]", "접촉저항[mOhm]", "출력전류 Irms[A]", "+/-초(63%)", "+/-초(98%)", "+/-초(37%)", "+/-저항", "+/-전류"] ("Array")
                        n88 = property class="Clust (strict)"(reference=w171) -> ("Controls[]"=w170:refnum<vi>[])  [unwired: 1 in, 2 out]
                        n89 = for {
                          tunnel: w170 -> [w173] mode=indexing
                          tunnel: w169 -> [w172] mode=indexing
                          n90 = property class="Ctl"(reference=w173, "DisabledEnum"=w172) -> ()  [unwired: 1 in, 2 out]
                        }
                      }
                    }
                  }
                  frame "저전압모드 동작검사" {
                    n91 = stacked-sequence {
                      seq-local: [w176 _ _] -> [_ w183 _]
                      tunnel: w175 -> [w177 w184 _]
                      tunnel: w174 -> [_ _ w193]
                      frame #0 {
                        n92 = property class="Clust (strict)"(reference=w177) -> ("Controls[]"=w180:refnum<vi>[])  [unwired: 1 in, 2 out]
                        n93 = Index Array(array=w180, index=0) -> (element=w181:refnum<vi>)
                        n94 = property class="Ctl"(reference=w181) -> ("Value"=w179:variant)  [unwired: 1 in, 2 out]
                        n95 = Variant To Data(type=T9."6.3.2 저온 작동/방치 시험" ("Test Mode"), Variant=w179) -> (data=w176:T9)  [unwired: 1 in, 1 out]
                      }
                      frame #1 {
                        n96 = property class="Clust (strict)"(reference=w184) -> ("Controls[]"=w186:refnum<vi>[])  [unwired: 1 in, 2 out]
                        n97 = case shown="\"6.3.2 저온 작동/방치 시험\", Default" w183 {
                          tunnel: [w189 w190] -> w185
                          frame "6.3.2 저온 작동/방치 시험", Default {
                            w189 = T15 [enum."Enabled", enum."Enabled", enum."Enabled", enum."Enabled", enum."Enabled", enum."Disabled and Grayed Out", enum."Enabled", enum."Enabled", enum."Enabled", enum."Enabled", enum."Enabled", enum."Enabled", enum."Enabled", enum."Enabled", enum."Enabled", enum."Enabled", enum."Enabled", enum."Enabled", enum."Enabled", enum."Disabled and Grayed Out", enum."Enabled", enum."Enabled"] items=["Enabled", "Disabled", "Disabled and Grayed Out"]  # 6.3.2, 6.3.3, 6.3.4, 6.3.8, 6.3.9
                          }
                          frame "6.3.6 온습도 싸이클 시험" {
                            w190 = T15 [enum."Enabled", enum."Enabled", enum."Enabled", enum."Enabled", enum."Enabled", enum."Enabled", enum."Enabled", enum."Enabled", enum."Enabled", enum."Enabled", enum."Enabled", enum."Enabled", enum."Enabled", enum."Enabled", enum."Enabled", enum."Enabled", enum."Enabled", enum."Enabled", enum."Enabled", enum."Disabled and Grayed Out", enum."Enabled", enum."Enabled"] items=["Enabled", "Disabled", "Disabled and Grayed Out"]  # 6.3.6
                          }
                        }
                        n98 = for {
                          tunnel: w186 -> [w188] mode=indexing
                          tunnel: w185 -> [w187] mode=indexing
                          n99 = property class="Ctl"(reference=w188, "DisabledEnum"=w187) -> ()  [unwired: 1 in, 2 out]
                        }
                      }
                      frame #2 {
                        w191 = T15 [enum."Disabled and Grayed Out", enum."Disabled and Grayed Out", enum."Disabled and Grayed Out", enum."Disabled and Grayed Out", enum."Enabled", enum."Disabled and Grayed Out", enum."Disabled and Grayed Out", enum."Disabled and Grayed Out", enum."Disabled and Grayed Out", enum."Enabled"] items=["Enabled", "Disabled", "Disabled and Grayed Out"]
                        n100 = property class="Clust (strict)"(reference=w193) -> ("Controls[]"=w192:refnum<vi>[])  [unwired: 1 in, 2 out]
                        n101 = for {
                          tunnel: w192 -> [w195] mode=indexing
                          tunnel: w191 -> [w194] mode=indexing
                          n102 = property class="Ctl"(reference=w195, "DisabledEnum"=w194) -> ()  [unwired: 1 in, 2 out]
                        }
                      }
                    }
                  }
                  frame "저전압모드 접촉저항" {
                    n103 = stacked-sequence {
                      seq-local: [w198 _ _] -> [_ w211 _]
                      tunnel: w197 -> [w204 w210 _]
                      tunnel: w196 -> [_ _ w218]
                      frame #0 {
                        n104 = property class="Clust (strict)"(reference=w204) -> ("Controls[]"=w201:refnum<vi>[])  [unwired: 1 in, 2 out]
                        n105 = disable-structure shown="Disabled" {
                          disable-tunnel: w201 -> [w205 _]
                          frame Disabled {
                            n106 = for {
                              tunnel: w205 -> [w207] mode=indexing
                              tunnel: [w206] -> _ mode=indexing
                              n107 = property class="Ctl"(reference=w207) -> ("Label.Text"=w206:string)  [unwired: 1 in, 2 out]
                            }
                          }
                          frame Enabled {
                          }
                        }
                        n108 = Index Array(array=w201, index=0) -> (element=w202:refnum<vi>)
                        n109 = property class="Ctl"(reference=w202) -> ("Value"=w200:variant)  [unwired: 1 in, 2 out]
                        n110 = Variant To Data(type=T9."6.3.2 저온 작동/방치 시험" ("Test Mode"), Variant=w200) -> (data=w198:T9)  [unwired: 1 in, 1 out]
                      }
                      frame #1 {
                        n111 = property class="Clust (strict)"(reference=w210) -> ("Controls[]"=w209:refnum<vi>[])  [unwired: 1 in, 2 out]
                        n112 = case shown="\"6.3.2 저온 작동/방치 시험\", Default" w211 {
                          tunnel: [w214 w215] -> w208
                          frame "6.3.2 저온 작동/방치 시험", Default {
                            w214 = T15 [enum."Enabled", enum."Enabled", enum."Enabled", enum."Enabled", enum."Enabled", enum."Disabled and Grayed Out", enum."Enabled", enum."Enabled", enum."Enabled", enum."Enabled", enum."Enabled", enum."Enabled", enum."Enabled", enum."Enabled", enum."Enabled", enum."Enabled", enum."Enabled", enum."Enabled", enum."Enabled", enum."Disabled and Grayed Out", enum."Enabled", enum."Enabled"] items=["Enabled", "Disabled", "Disabled and Grayed Out"]  # 6.3.2, 6.3.3, 6.3.4, 6.3.8, 6.3.9
                          }
                          frame "6.3.6 온습도 싸이클 시험" {
                            w215 = T15 [enum."Enabled", enum."Enabled", enum."Enabled", enum."Enabled", enum."Enabled", enum."Enabled", enum."Enabled", enum."Enabled", enum."Enabled", enum."Enabled", enum."Enabled", enum."Enabled", enum."Enabled", enum."Enabled", enum."Enabled", enum."Enabled", enum."Enabled", enum."Enabled", enum."Enabled", enum."Disabled and Grayed Out", enum."Enabled", enum."Enabled"] items=["Enabled", "Disabled", "Disabled and Grayed Out"]  # 6.3.6
                          }
                        }
                        n113 = for {
                          tunnel: w209 -> [w213] mode=indexing
                          tunnel: w208 -> [w212] mode=indexing
                          n114 = property class="Ctl"(reference=w213, "DisabledEnum"=w212) -> ()  [unwired: 1 in, 2 out]
                        }
                      }
                      frame #2 {
                        w216 = T15 [enum."Disabled and Grayed Out", enum."Disabled and Grayed Out", enum."Disabled and Grayed Out", enum."Enabled", enum."Disabled and Grayed Out", enum."Disabled and Grayed Out", enum."Disabled and Grayed Out", enum."Disabled and Grayed Out", enum."Enabled", enum."Disabled and Grayed Out"] items=["Enabled", "Disabled", "Disabled and Grayed Out"]
                        (unwired) string[] ["전압 63%[초]", "전압 98%[초]", "전류 37%[초]", "접촉저항[mOhm]", "출력전류 Irms[A]", "+/-초(63%)", "+/-초(98%)", "+/-초(37%)", "+/-저항", "+/-전류"] ("Array")
                        n115 = property class="Clust (strict)"(reference=w218) -> ("Controls[]"=w217:refnum<vi>[])  [unwired: 1 in, 2 out]
                        n116 = for {
                          tunnel: w217 -> [w220] mode=indexing
                          tunnel: w216 -> [w219] mode=indexing
                          n117 = property class="Ctl"(reference=w220, "DisabledEnum"=w219) -> ()  [unwired: 1 in, 2 out]
                        }
                      }
                    }
                  }
                  frame "고전압모드 동작검사" {
                    n118 = stacked-sequence {
                      seq-local: [w223 _ _] -> [_ w231 _]
                      tunnel: w222 -> [w224 w230 _]
                      tunnel: w221 -> [_ _ w240]
                      frame #0 {
                        n119 = property class="Clust (strict)"(reference=w224) -> ("Controls[]"=w227:refnum<vi>[])  [unwired: 1 in, 2 out]
                        n120 = Index Array(array=w227, index=0) -> (element=w228:refnum<vi>)
                        n121 = property class="Ctl"(reference=w228) -> ("Value"=w226:variant)  [unwired: 1 in, 2 out]
                        n122 = Variant To Data(type=T9."6.3.2 저온 작동/방치 시험" ("Test Mode"), Variant=w226) -> (data=w223:T9)  [unwired: 1 in, 1 out]
                      }
                      frame #1 {
                        n123 = property class="Clust (strict)"(reference=w230) -> ("Controls[]"=w233:refnum<vi>[])  [unwired: 1 in, 2 out]
                        n124 = case shown="\"6.3.6 온습도 싸이클 시험\"" w231 {
                          tunnel: [w236 w237] -> w232
                          frame "6.3.2 저온 작동/방치 시험", Default {
                            w236 = T15 [enum."Enabled", enum."Enabled", enum."Enabled", enum."Enabled", enum."Enabled", enum."Disabled and Grayed Out", enum."Enabled", enum."Enabled", enum."Enabled", enum."Enabled", enum."Enabled", enum."Enabled", enum."Enabled", enum."Enabled", enum."Enabled", enum."Enabled", enum."Enabled", enum."Enabled", enum."Enabled", enum."Enabled", enum."Enabled", enum."Enabled"] items=["Enabled", "Disabled", "Disabled and Grayed Out"]  # 6.3.2, 6.3.3, 6.3.4, 6.3.8, 6.3.9
                          }
                          frame "6.3.6 온습도 싸이클 시험" {
                            w237 = T15 [enum."Enabled", enum."Enabled", enum."Enabled", enum."Enabled", enum."Enabled", enum."Enabled", enum."Enabled", enum."Enabled", enum."Enabled", enum."Enabled", enum."Enabled", enum."Enabled", enum."Enabled", enum."Enabled", enum."Enabled", enum."Enabled", enum."Enabled", enum."Enabled", enum."Enabled", enum."Enabled", enum."Enabled", enum."Enabled"] items=["Enabled", "Disabled", "Disabled and Grayed Out"]  # 6.3.6
                          }
                        }
                        n125 = for {
                          tunnel: w233 -> [w235] mode=indexing
                          tunnel: w232 -> [w234] mode=indexing
                          n126 = property class="Ctl"(reference=w235, "DisabledEnum"=w234) -> ()  [unwired: 1 in, 2 out]
                        }
                      }
                      frame #2 {
                        w238 = T15 [enum."Enabled", enum."Enabled", enum."Enabled", enum."Enabled", enum."Enabled", enum."Enabled", enum."Enabled", enum."Enabled", enum."Enabled", enum."Enabled"] items=["Enabled", "Disabled", "Disabled and Grayed Out"]
                        (unwired) string[] ["전압 63%[초]", "전압 98%[초]", "전류 37%[초]", "접촉저항[mOhm]", "출력전류 Irms[A]", "+/-초(63%)", "+/-초(98%)", "+/-초(37%)", "+/-저항", "+/-전류"] ("Array")
                        n127 = property class="Clust (strict)"(reference=w240) -> ("Controls[]"=w239:refnum<vi>[])  [unwired: 1 in, 2 out]
                        n128 = for {
                          tunnel: w239 -> [w242] mode=indexing
                          tunnel: w238 -> [w241] mode=indexing
                          n129 = property class="Ctl"(reference=w242, "DisabledEnum"=w241) -> ()  [unwired: 1 in, 2 out]
                        }
                      }
                    }
                  }
                }
              }
              frame Enabled {
                n130 = call "TestModeUpdate.vi"("Update?"=TRUE) -> ()  [unwired: 9 in, 2 out]
              }
            }
          }
          frame #2 {
            n131 = call "fgv_rc-config.vi"("cmd"=rw."read") -> ("Testconfig out"=w255:T3)  [unwired: 9 in, 1 out]
            n132 = Unbundle By Name(w255) -> ("Freq"=w250:dbl, "level[V]"=w251:dbl, "duty"=w252:dbl, "ON time[ms]"=w253:dbl, "Record Len"=w254:i32, "Time Div"=w244:u16)
            n133 = disable-structure shown="Disabled" {
              disable-tunnel: w244 -> [w256 _]
              frame Disabled {
                w257 = u16[] [10, 20, 50, 100, 200, 500, 1000, 2000] items=["10m"=10, "20ms"=20, "50ms"=50, "100ms"=100, "200ms"=200, "500ms"=500, "1s"=1000, "2s"=2000]
                n134 = Index Array(array=w257, index=w256) -> ()  [unwired: 1 out]
              }
              frame Enabled {
              }
            }
            n135 = Bundle By Name(cluster=cluster{"Record Len":i32, "Time Div":u16} {"Record Len"=4, "Time Div"=100} ("Oscilloscope_rc"), "Record Len"=w254, "Time Div"=w244) -> (w245:cluster{"Record Len":i32, "Time Div":u16})
            n136 = Bundle(cluster=T10 {"Freq"=1.0, "level[V]"=12.0, "duty"=20.0, "On time[ms]"=500.0} ("Control Signal_rc"), "Freq"=w250, "level[V]"=w251, "duty"=w252, "On time[ms]"=w253) -> (w246:T10)
            n137 = global write "Glob_Ref.vi" "Control Signal_HV"(w246) -> ()
            n138 = global write "Glob_Ref.vi" "Control Signal_LCR"(w246) -> ()
            n139 = global write "Glob_Ref.vi" "Control Signal_LV"(w246) -> ()
            n140 = global write "Glob_Ref.vi" "Control Signal_res"(w246) -> ()
            n141 = global write "Glob_Ref.vi" "Control Signal_rc"(w246) -> ()
            n142 = global write "Glob_Ref.vi" "Control Signal_B1"(w246) -> ()
            n143 = global write "Glob_Ref.vi" "Control Signal_B2"(w246) -> ()
            n144 = global write "Glob_Ref.vi" "Control Signal_B3"(w246) -> ()
            n145 = global write "Glob_Ref.vi" "Oscilloscope_res"(w245) -> ()
            n146 = global write "Glob_Ref.vi" "Oscilloscope_rc"(w245) -> ()
            n147 = global write "Glob_Ref.vi" "Oscilloscope_B1"(w245) -> ()
            n148 = global write "Glob_Ref.vi" "Oscilloscope_B2"(w245) -> ()
            n149 = global write "Glob_Ref.vi" "Oscilloscope_B3"(w245) -> ()
            n150 = global write "Glob_Ref.vi" "Oscilloscope_HV"(w245) -> ()
            n151 = global write "Glob_Ref.vi" "Oscilloscope_LCR"(w245) -> ()
            n152 = global write "Glob_Ref.vi" "Oscilloscope_LV"(w245) -> ()
          }
        }
      }
    }
  }
  n153 = global write "Global_params.vi" "TestConditons"(w1) -> ()
